vi "LSMcontroller_v64_updatedwaveformhandling.vi"() -> ()   [LabVIEW 2015] (continued)
                                frame False {
                                }
                                frame True {
                                n2579 = local write "set as Rp?"(FALSE ("set as Rp?")) -> ()
                                }
                              }
                            }
                          }
                        }
                        frame True {
                        }
                      }
                      n2580 = local read "sealtest"() -> (w5565:bool)
                      n2581 = Not(x=w5565) -> (.not. x?=w5564:bool)
                    }
                  }
                  frame #4 {
                    n2582 = call "tempconfigAO.vi"("command"="get") -> ("Temp Config out"=w5735:T25)  [unwired: 1 in]
                    n2583 = Unbundle By Name(w5735) -> ("AO"=w5734:refnum<k21>[], "E_AO"=w5733:errorcluster[])
                    n2584 = call "configuration.vi"("command"="get") -> ("config out"=w5716:T11)  [unwired: 2 in, 1 out]
                    n2585 = call "tempconfigAI.vi"("command"="get") -> ("Temp Config out"=w5722:T26)  [unwired: 1 in]
                    n2586 = Unbundle By Name(w5716) -> ("Device 1 sampleclock out"=w5713:tag, "Device 1 Starttrigger out"=w5712:tag)
                    n2587 = Unbundle By Name(w5722) -> ("AI"=w5723:refnum<k21>, "E_AI"=w5724:errorcluster)
                    n2588 = for {
                      tunnel: w5734 -> [w5739] mode=indexing
                      tunnel: w5733 -> [w5738] mode=indexing
                      tunnel: [w5737] -> w5729 mode=indexing
                      n2589 = call <vilib>:"DAQmx Stop Task.vi"("task/channels in"=w5739, "error in"=w5738) -> ("task out"=w5740:refnum<k21>, "error out"=w5741:errorcluster)  [unwired: 12 in]
                      n2590 = call <vilib>:"DAQmx Clear Task.vi"("task in"=w5740, "error in"=w5741) -> ("error out"=w5737:errorcluster)  [unwired: 13 in]
                    }
                    n2591 = call <vilib>:"DAQmx Stop Task.vi"("task/channels in"=w5723, "error in"=w5724) -> ("task out"=w5720:refnum<k21>, "error out"=w5719:errorcluster)  [unwired: 12 in]
                    n2592 = call <vilib>:"DAQmx Disconnect Terminals.vi"("source terminal"=tag "/Dev1/ai/SampleClock", "destination terminal"=w5713) -> ("error out"=w5710:errorcluster)  [unwired: 13 in]
                    n2593 = call <vilib>:"DAQmx Clear Task.vi"("task in"=w5720, "error in"=w5719) -> ("error out"=w5718:errorcluster)  [unwired: 13 in]
                    n2594 = call "tempconfigAO.vi"("command"="get") -> ("Temp Config out"=w5730:T25)  [unwired: 1 in]
                    n2595 = Bundle By Name(cluster=w5730, "E_AO"=w5729) -> (w5728:T25)
                    n2596 = call "tempconfigAI.vi"("command"="get") -> ("Temp Config out"=w5726:T26)  [unwired: 1 in]
                    n2597 = Bundle By Name(cluster=w5726, "E_AI"=w5718) -> (w5717:T26)
                    n2598 = call "tempconfigAO.vi"("Temp Config in"=w5728, "command"="set") -> ()  [unwired: 1 out]
                    n2599 = call <vilib>:"DAQmx Disconnect Terminals.vi"("source terminal"=tag "/Dev1/ai/StartTrigger", "destination terminal"=w5712, "error in"=w5710) -> ()  [unwired: 12 in, 1 out]
                    n2600 = call "tempconfigAI.vi"("Temp Config in"=w5717, "command"="set") -> ()  [unwired: 1 out]
                  }
                  frame #5 {
                    w5744 = T21 4 items=["no dialog", "OK message", "continue or stop message", "OK message + warnings", "continue/stop + warnings"] ("type of dialog (OK msg:1)")
                    n2601 = call "displayerrors.vi"() -> ("error IO"=w5743:errorcluster)
                    n2602 = call "zeropatch.vi"() -> ()  [unwired: 12 in]
                    n2603 = call <vilib>:"Simple Error Handler.vi"("type of dialog (OK msg:1)"=w5744, "error in (no error)"=w5743) -> ("error out"=w5742:errorcluster)  [unwired: 3 in, 4 out]
                    n2604 = call <vilib>:"Clear Errors.vi"("error in (no error)"=w5742) -> ()  [unwired: 5 in, 2 out]
                  }
                }
              }
            }
          }
          event "readpatch": Value Change {
            n2605 = event-data() -> ()  [unwired: 1 in, 6 out]
            n2606 = local read "readpatch"() -> (w5745:bool)
            n2607 = case shown="True" w5745 {
              frame False {
              }
              frame True {
                n2608 = stacked-sequence {
                  seq-local: [w5746 _ _ _ _ _] -> [_ w5779 _ w5831 _ _]
                  frame #0 {
                    n2609 = stacked-sequence {
                      tunnel: [_ w5758 _] -> w5746
                      frame #0 {
                        n2610 = call "2pparameters.vi"("command"="get") -> ("params out"=w5751:T10)  [unwired: 1 in]
                        n2611 = Unbundle By Name(w5751) -> ("autoshutter"=w5752:bool)
                        n2612 = local read "OCchecked?"() -> (w5749:bool)
                        n2613 = call "sealtestwfparams.vi"("command"="set") -> ()  [unwired: 6 in, 1 out]
                        n2614 = case shown="False" w5749 {
                          frame False {
                            n2615 = One Button Dialog(message="Is the OC gain correct?", button name ("OK")="ok") -> (true=w5753:bool)
                            n2616 = local write "OCchecked?"(w5753) -> ()
                          }
                          frame True {
                          }
                        }
                        n2617 = case shown="True" w5752 {
                          frame False {
                          }
                          frame True {
                            n2618 = call "shuttercontrol.vi"("command"="close") -> ()  [unwired: 1 in, 1 out]
                          }
                        }
                        n2619 = call "allAI-temp.vi"("command"=enum16{"get", "set", "clear", "append"}."clear") -> ()  [unwired: 3 in, 2 out]
                      }
                      frame #1 {
                        n2620 = call "sealtestwfparams.vi"("command"="get") -> ("Params out"=w5764:T22)  [unwired: 6 in]
                        n2621 = Unbundle By Name(w5764) -> ("AO parameters"=w5762:T23)
                        n2622 = Index Array(array=w5762, index=1) -> (element=w5761:T24)
                        n2623 = call "generateRampedSquareWave_fromAOparameters.vi"("AO params"=w5761) -> ("Waveform"=w5757:waveform(dbl), "wflength"=w5758:i32)
                        n2624 = Build Array(w5757) -> (w5760:waveform(dbl)[])
                        n2625 = call "waveformssealtestbuffer.vi"("AO wf in"=w5760, "command"="set") -> ()  [unwired: 1 out]
                      }
                      frame #2 {
                        n2626 = local read "Vholding (mV)"() -> (w5767:sgl)
                        n2627 = local read "Current Clamp"() -> (w5773:bool)
                        n2628 = local read "Voltage Clamp"() -> (w5772:bool)
                        n2629 = local read "OCgain"() -> (w5768:sgl)
                        n2630 = local read "CC_ICgain"() -> (w5771:dbl)
                        n2631 = local read "holdon"() -> (w5766:bool)
                        n2632 = call "patchparameters.vi"("command"="get") -> ("Params out"=w5775:T13)  [unwired: 1 in]
                        n2633 = Bundle By Name(cluster=w5775, "VC"=w5772, "CC"=w5773, "CC_icg (pA/mv)"=w5771, "VC_icg (mV/mV)"=10.0, "OCG (mV/pA)"=w5768, "OVG (mV/mV)"=0.1, "Vhold (mV)"=w5767, "holdon"=w5766) -> (w5774:T13)
                        n2634 = call "patchparameters.vi"("Params in"=w5774, "command"="set") -> ()  [unwired: 1 out]
                      }
                    }
                  }
                  frame #1 {
                    w5778 = 2
                    n2635 = call "patchparameters.vi"("command"="get") -> ("Params out"=w5786:T13)  [unwired: 1 in]
                    n2636 = Unbundle By Name(w5786) -> ("holdon"=w5785:bool, "Vhold (mV)"=w5784:sgl, "CC_icg (pA/mv)"=w5792:sgl, "CC"=w5790:bool, "VC_icg (mV/mV)"=w5791:sgl)
                    n2637 = Select(t=w5792, s=w5790, f=w5791) -> (s? t:f=w5793:sgl)
                    n2638 = To Single Precision Float(number=0.001 ("y")) -> (single precision float=w5794:sgl)
                    n2639 = Compound Arithmetic op=MULTIPLY(w5784, w5793, w5794) -> (w5788:sgl)
                    n2640 = case shown="False" w5785 {
                      tunnel: w5788 -> [_ w5806]
                      tunnel: [0.0 w5806] -> w5781
                      frame False {
                      }
                      frame True {
                      }
                    }
                    n2641 = Greater Than 0?(x=w5778) -> (x > 0?=w5780:bool)
                    n2642 = case shown="True" w5780 {
                      tunnel: w5779 -> [_ w5795]
                      tunnel: w5778 -> [_ w5798]
                      frame False {
                      }
                      frame True {
                        n2643 = Initialize Array(sgl 0.0 ("element"), w5798, w5795) -> (w5796:sgl[][])
                        n2644 = call "allAI-temp.vi"("array in"=w5796, "command"=enum16{"get", "set", "clear", "append"}."set") -> ()  [unwired: 2 in, 2 out]
                      }
                    }
                    n2645 = flat-sequence {
                      tunnel: w5779 -> [w5802]
                      tunnel: w5779 -> [w5801]
                      tunnel: [w5801] -> w5783
                      tunnel: [w5800] -> w5782
                      tunnel: w5781 -> [w5800]
                      tunnel: w5783 -> [w5804]
                      tunnel: w5782 -> [w5803]
                      frame #0 {
                        n2646 = call "prepAI_sealtest.vi"("samples per channel"=w5802) -> ()  [unwired: 2 in]
                      }
                      frame #1 {
                        n2647 = call "prepAO_sealtest.vi"("Vhold"=w5803, "samples per channel"=w5804) -> ()  [unwired: 1 in]
                      }
                    }
                  }
                  frame #2 {
                    n2648 = stacked-sequence {
                      frame #0 {
                        n2649 = call "tempconfigAO.vi"("command"="get") -> ("Temp Config out"=w5810:T25)  [unwired: 1 in]
                        n2650 = Unbundle By Name(w5810) -> ("AO"=w5811:refnum<k21>[], "E_AO"=w5812:errorcluster[])
                        n2651 = for {
                          tunnel: w5811 -> [w5820] mode=indexing
                          tunnel: w5812 -> [w5819] mode=indexing
                          tunnel: [w5818] -> w5814 mode=indexing
                          tunnel: [w5817] -> w5815 mode=indexing
                          n2652 = call <vilib>:"DAQmx Start Task.vi"("task/channels in"=w5820, "error in"=w5819) -> ("task out"=w5818:refnum<k21>, "error out"=w5817:errorcluster)  [unwired: 12 in]
                        }
                        n2653 = call "tempconfigAO.vi"("command"="get") -> ("Temp Config out"=w5813:T25)  [unwired: 1 in]
                        n2654 = Bundle By Name(cluster=w5813, "AO"=w5814, "E_AO"=w5815) -> (w5816:T25)
                        n2655 = call "tempconfigAO.vi"("Temp Config in"=w5816, "command"="set") -> ()  [unwired: 1 out]
                      }
                      frame #1 {
                        n2656 = call "tempconfigAI.vi"("command"="get") -> ("Temp Config out"=w5822:T26)  [unwired: 1 in]
                        n2657 = Unbundle By Name(w5822) -> ("AI"=w5827:refnum<k21>, "E_AI"=w5828:errorcluster)
                        n2658 = call <vilib>:"DAQmx Start Task.vi"("task/channels in"=w5827, "error in"=w5828) -> ("task out"=w5829:refnum<k21>, "error out"=w5830:errorcluster)  [unwired: 12 in]
                        n2659 = call "tempconfigAI.vi"("command"="get") -> ("Temp Config out"=w5824:T26)  [unwired: 1 in]
                        n2660 = Bundle By Name(cluster=w5824, "AI"=w5829, "E_AI"=w5830) -> (w5826:T26)
                        n2661 = call "tempconfigAI.vi"("Temp Config in"=w5826, "command"="set") -> ()  [unwired: 1 out]
                      }
                    }
                  }
                  frame #3 {
                    n2662 = while {
                      tunnel: w5831 -> [w5832]
                      stop <- w5833 stop-if-true
                      n2663 = local read "readpatch"() -> (w5836:bool)
                      n2664 = Not(x=w5836) -> (.not. x?=w5835:bool)
                      n2665 = case shown="True" w5835 {
                        tunnel: w5832 -> [w5837 _]
                        frame False {
                          n2666 = stacked-sequence {
                            seq-local: [w5838 _ _ _ _ _] -> [_ w5847 _ w5870 w5917 w5936]
                            tunnel: w5837 -> [_ _ w5855 _ w5916 _]
                            frame #0 {
                              n2667 = call "patchparameters.vi"("command"="get") -> ("Params out"=w5845:T13)  [unwired: 1 in]
                              n2668 = local read "Vholding (mV)"() -> (w5842:sgl)
                              n2669 = Unbundle By Name(w5845) -> ("Vhold (mV)"=w5841:sgl, "holdon"=w5844:bool)
                              n2670 = local read "holdon"() -> (w5843:bool)
                              n2671 = Not Equal?(x=w5842, y=w5841) -> (x != y?=w5840:bool)
                              n2672 = Not Equal?(x=w5844, y=w5843) -> (x != y?=w5839:bool)
                              n2673 = Or(x=w5840, y=w5839) -> (x .or. y?=w5838:bool)
                            }
                            frame #1 {
                              n2674 = case shown="False" w5847 {
                                frame False {
                                }
                                frame True {
                                n2675 = local read "Vholding (mV)"() -> (w5850:sgl)
                                n2676 = local read "holdon"() -> (w5848:bool)
                                n2677 = call "patchparameters.vi"("command"="get") -> ("Params out"=w5851:T13)  [unwired: 1 in]
                                n2678 = Bundle By Name(cluster=w5851, "Vhold (mV)"=w5850, "holdon"=w5848) -> (w5849:T13)
                                n2679 = call "patchparameters.vi"("Params in"=w5849, "command"="set") -> ()  [unwired: 1 out]
                                }
                              }
                            }
                            frame #2 {
                              n2680 = call "tempconfigAI.vi"("command"="get") -> ("Temp Config out"=w5865:T26)  [unwired: 1 in]
                              n2681 = Unbundle By Name(w5865) -> ("AI"=w5864:refnum<k21>, "E_AI"=w5863:errorcluster)
                              n2682 = call-poly <vilib>:"DAQmx Read.vi"("task/channels in"=w5864, "number of samples per channel"=w5855, "timeout"=10.0, "error in"=w5863) -> ("task out"=w5859:refnum<k21>, "data"=w5856:i16[][], "error out"=w5868:errorcluster)  [unwired: 9 in]
                              n2683 = call "tempconfigAI.vi"("command"="get") -> ("Temp Config out"=w5860:T26)  [unwired: 1 in]
                              n2684 = Bundle By Name(cluster=w5860, "AI"=w5859, "E_AI"=w5868) -> (w5867:T26)
                              n2685 = To Single Precision Float(number=w5856) -> (single precision float=w5858:sgl[][])
                              n2686 = call "tempconfigAI.vi"("Temp Config in"=w5867, "command"="set") -> ()  [unwired: 1 out]
                              n2687 = call "allAI-temp.vi"("array in"=w5858, "command"=enum16{"get", "set", "clear", "append"}."set") -> ()  [unwired: 2 in, 2 out]
                            }
                            frame #3 {
                              n2688 = case shown="True" w5870 {
                                frame False {
                                }
                                frame True {
                                n2689 = call "tempconfigAO.vi"("command"="get") -> ("Temp Config out"=w5909:T25)  [unwired: 1 in]
                                n2690 = Unbundle By Name(w5909) -> ("AO"=w5908:refnum<k21>[], "E_AO"=w5907:errorcluster[])
                                n2691 = call "tempconfigAI.vi"("command"="get") -> ("Temp Config out"=w5896:T26)  [unwired: 1 in]
                                n2692 = Unbundle By Name(w5896) -> ("AI"=w5897:refnum<k21>, "E_AI"=w5898:errorcluster)
                                n2693 = for {
                                tunnel: w5908 -> [w5913] mode=indexing
                                tunnel: w5907 -> [w5912] mode=indexing
                                tunnel: [w5911] -> w5903 mode=indexing
                                n2694 = call <vilib>:"DAQmx Stop Task.vi"("task/channels in"=w5913, "error in"=w5912) -> ("task out"=w5914:refnum<k21>, "error out"=w5915:errorcluster)  [unwired: 12 in]
                                n2695 = call <vilib>:"DAQmx Clear Task.vi"("task in"=w5914, "error in"=w5915) -> ("error out"=w5911:errorcluster)  [unwired: 13 in]
                                }
                                n2696 = call <vilib>:"DAQmx Stop Task.vi"("task/channels in"=w5897, "error in"=w5898) -> ("task out"=w5894:refnum<k21>, "error out"=w5893:errorcluster)  [unwired: 12 in]
                                n2697 = call <vilib>:"DAQmx Clear Task.vi"("task in"=w5894, "error in"=w5893) -> ("error out"=w5892:errorcluster)  [unwired: 13 in]
                                n2698 = call "tempconfigAO.vi"("command"="get") -> ("Temp Config out"=w5904:T25)  [unwired: 1 in]
                                n2699 = Bundle By Name(cluster=w5904, "E_AO"=w5903) -> (w5902:T25)
                                n2700 = call "tempconfigAI.vi"("command"="get") -> ("Temp Config out"=w5900:T26)  [unwired: 1 in]
                                n2701 = Bundle By Name(cluster=w5900, "E_AI"=w5892) -> (w5891:T26)
                                n2702 = call "tempconfigAO.vi"("Temp Config in"=w5902, "command"="set") -> ()  [unwired: 1 out]
                                n2703 = call "tempconfigAI.vi"("Temp Config in"=w5891, "command"="set") -> ()  [unwired: 1 out]
                                }
                              }
                              n2704 = call "allAI-temp.vi"("command"=enum16{"get", "set", "clear", "append"}."get") -> ("array out"=w5874:sgl[][])  [unwired: 3 in, 1 out]
                              n2705 = call "tempconfigAI.vi"("command"="get") -> ("Temp Config out"=w5886:T26)  [unwired: 1 in]
                              n2706 = call "tempconfigAI.vi"("command"="get") -> ("Temp Config out"=w5888:T26)  [unwired: 1 in]
                              n2707 = Unbundle By Name(w5886) -> ("header"=w5884:dbl[])
                              n2708 = Unbundle By Name(w5888) -> ("header"=w5890:dbl[])
                              n2709 = Index Array(array=w5874, index (row) #1=1 ("index (row)"), index (row) #2=0 ("index (row)")) -> (element #1=w5872:sgl[], element #2=w5871:sgl[])  [unwired: 2 in]
                              n2710 = local read "OCgain"() -> (w5878:sgl)
                              n2711 = call "Unscaledtoscaled.vi"("Unscaled Data"=w5872, "Header Information"=w5884) -> ("Array"=w5883:sgl[])  [unwired: 1 in]
                              n2712 = call "Unscaledtoscaled.vi"("Unscaled Data"=w5871, "Header Information"=w5890) -> ("Array"=w5887:sgl[])  [unwired: 1 in]
                              n2713 = Multiply(x=w5883, y=0.1) -> (x*y=w5880:dbl[])
                              n2714 = Divide(x=w5887, y=w5878) -> (x/y=w5879:sgl[])
                              n2715 = Build Array(w5880, w5879) -> (w5882:dbl[][])
                              n2716 = Multiply(x=w5882, y=1000.0) -> (x*y=w5869:dbl[][])
                              n2717 = local write "Patch readout"(w5869) -> ()
                            }
                            frame #4 {
                              n2718 = case shown="True" w5917 {
                                tunnel: w5916 -> [_ w5918]
                                frame False {
                                }
                                frame True {
                                n2719 = call "patchparameters.vi"("command"="get") -> ("Params out"=w5922:T13)  [unwired: 1 in]
                                n2720 = Unbundle By Name(w5922) -> ("holdon"=w5921:bool, "Vhold (mV)"=w5920:sgl, "CC_icg (pA/mv)"=w5928:sgl, "CC"=w5926:bool, "VC_icg (mV/mV)"=w5927:sgl)
                                n2721 = Select(t=w5928, s=w5926, f=w5927) -> (s? t:f=w5929:sgl)
                                n2722 = To Single Precision Float(number=0.001 ("y")) -> (single precision float=w5930:sgl)
                                n2723 = Compound Arithmetic op=MULTIPLY(w5920, w5929, w5930) -> (w5924:sgl)
                                n2724 = case shown="True" w5921 {
                                tunnel: w5924 -> [_ w5935]
                                tunnel: [0.0 w5935] -> w5919
                                frame False {
                                }
                                frame True {
                                }
                                }
                                n2725 = flat-sequence {
                                tunnel: w5918 -> [w5931]
                                tunnel: w5919 -> [w5933]
                                tunnel: w5918 -> [w5932]
                                frame #0 {
                                n2726 = call "prepAI_sealtest.vi"("samples per channel"=w5931) -> ()  [unwired: 2 in]
                                }
                                frame #1 {
                                n2727 = call "prepAO_sealtest.vi"("Vhold"=w5933, "samples per channel"=w5932) -> ()  [unwired: 1 in]
                                }
                                }
                                }
                              }
                            }
                            frame #5 {
                              n2728 = case shown="True" w5936 {
                                frame False {
                                }
                                frame True {
                                n2729 = stacked-sequence {
                                frame #0 {
                                n2730 = call "tempconfigAO.vi"("command"="get") -> ("Temp Config out"=w5943:T25)  [unwired: 1 in]
                                n2731 = Unbundle By Name(w5943) -> ("AO"=w5942:refnum<k21>[], "E_AO"=w5941:errorcluster[])
                                n2732 = for {
                                tunnel: w5942 -> [w5950] mode=indexing
                                tunnel: w5941 -> [w5949] mode=indexing
                                tunnel: [w5948] -> w5939 mode=indexing
                                tunnel: [w5947] -> w5938 mode=indexing
                                n2733 = call <vilib>:"DAQmx Start Task.vi"("task/channels in"=w5950, "error in"=w5949) -> ("task out"=w5948:refnum<k21>, "error out"=w5947:errorcluster)  [unwired: 12 in]
                                }
                                n2734 = call "tempconfigAO.vi"("command"="get") -> ("Temp Config out"=w5940:T25)  [unwired: 1 in]
                                n2735 = Bundle By Name(cluster=w5940, "AO"=w5939, "E_AO"=w5938) -> (w5937:T25)
                                n2736 = call "tempconfigAO.vi"("Temp Config in"=w5937, "command"="set") -> ()  [unwired: 1 out]
                                }
                                frame #1 {
                                n2737 = call "tempconfigAI.vi"("command"="get") -> ("Temp Config out"=w5952:T26)  [unwired: 1 in]
                                n2738 = Unbundle By Name(w5952) -> ("AI"=w5957:refnum<k21>, "E_AI"=w5958:errorcluster)
                                n2739 = call <vilib>:"DAQmx Start Task.vi"("task/channels in"=w5957, "error in"=w5958) -> ("task out"=w5959:refnum<k21>, "error out"=w5960:errorcluster)  [unwired: 12 in]
                                n2740 = call "tempconfigAI.vi"("command"="get") -> ("Temp Config out"=w5954:T26)  [unwired: 1 in]
                                n2741 = Bundle By Name(cluster=w5954, "AI"=w5959, "E_AI"=w5960) -> (w5956:T26)
                                n2742 = call "tempconfigAI.vi"("Temp Config in"=w5956, "command"="set") -> ()  [unwired: 1 out]
                                }
                                }
                                }
                              }
                            }
                          }
                        }
                        frame True {
                        }
                      }
                      n2743 = local read "readpatch"() -> (w5834:bool)
                      n2744 = Not(x=w5834) -> (.not. x?=w5833:bool)
                    }
                  }
                  frame #4 {
                    n2745 = call "tempconfigAO.vi"("command"="get") -> ("Temp Config out"=w5986:T25)  [unwired: 1 in]
                    n2746 = Unbundle By Name(w5986) -> ("AO"=w5985:refnum<k21>[], "E_AO"=w5984:errorcluster[])
                    n2747 = call "configuration.vi"("command"="get") -> ("config out"=w5967:T11)  [unwired: 2 in, 1 out]
                    n2748 = call "tempconfigAI.vi"("command"="get") -> ("Temp Config out"=w5973:T26)  [unwired: 1 in]
                    n2749 = Unbundle By Name(w5967) -> ("Device 1 sampleclock out"=w5964:tag, "Device 1 Starttrigger out"=w5963:tag)
                    n2750 = Unbundle By Name(w5973) -> ("AI"=w5974:refnum<k21>, "E_AI"=w5975:errorcluster)
                    n2751 = for {
                      tunnel: w5985 -> [w5990] mode=indexing
                      tunnel: w5984 -> [w5989] mode=indexing
                      tunnel: [w5988] -> w5980 mode=indexing
                      n2752 = call <vilib>:"DAQmx Stop Task.vi"("task/channels in"=w5990, "error in"=w5989) -> ("task out"=w5991:refnum<k21>, "error out"=w5992:errorcluster)  [unwired: 12 in]
                      n2753 = call <vilib>:"DAQmx Clear Task.vi"("task in"=w5991, "error in"=w5992) -> ("error out"=w5988:errorcluster)  [unwired: 13 in]
                    }
                    n2754 = call <vilib>:"DAQmx Stop Task.vi"("task/channels in"=w5974, "error in"=w5975) -> ("task out"=w5971:refnum<k21>, "error out"=w5970:errorcluster)  [unwired: 12 in]
                    n2755 = call <vilib>:"DAQmx Disconnect Terminals.vi"("source terminal"=tag "/Dev1/ai/SampleClock", "destination terminal"=w5964) -> ("error out"=w5961:errorcluster)  [unwired: 13 in]
                    n2756 = call <vilib>:"DAQmx Clear Task.vi"("task in"=w5971, "error in"=w5970) -> ("error out"=w5969:errorcluster)  [unwired: 13 in]
                    n2757 = call "tempconfigAO.vi"("command"="get") -> ("Temp Config out"=w5981:T25)  [unwired: 1 in]
                    n2758 = Bundle By Name(cluster=w5981, "E_AO"=w5980) -> (w5979:T25)
                    n2759 = call "tempconfigAI.vi"("command"="get") -> ("Temp Config out"=w5977:T26)  [unwired: 1 in]
                    n2760 = Bundle By Name(cluster=w5977, "E_AI"=w5969) -> (w5968:T26)
                    n2761 = call "tempconfigAO.vi"("Temp Config in"=w5979, "command"="set") -> ()  [unwired: 1 out]
                    n2762 = call <vilib>:"DAQmx Disconnect Terminals.vi"("source terminal"=tag "/Dev1/ai/StartTrigger", "destination terminal"=w5963, "error in"=w5961) -> ()  [unwired: 12 in, 1 out]
                    n2763 = call "tempconfigAI.vi"("Temp Config in"=w5968, "command"="set") -> ()  [unwired: 1 out]
                  }
                  frame #5 {
                    w5995 = T21 4 items=["no dialog", "OK message", "continue or stop message", "OK message + warnings", "continue/stop + warnings"] ("type of dialog (OK msg:1)")
                    n2764 = call "displayerrors.vi"() -> ("error IO"=w5994:errorcluster)
                    n2765 = call "zeropatch.vi"() -> ()  [unwired: 12 in]
                    n2766 = call <vilib>:"Simple Error Handler.vi"("type of dialog (OK msg:1)"=w5995, "error in (no error)"=w5994) -> ("error out"=w5993:errorcluster)  [unwired: 3 in, 4 out]
                    n2767 = call <vilib>:"Clear Errors.vi"("error in (no error)"=w5993) -> ()  [unwired: 5 in, 2 out]
                  }
                }
              }
            }
          }
          event "Current Clamp": Value Change {
            n2768 = event-data() -> ()  [unwired: 1 in, 6 out]
            n2769 = local read "Current Clamp"() -> (w6000:bool)
            n2770 = property on="Vholding (mV)" class="DigNum (strict)"("Caption.Text"="Ihold (pA)") -> ()  [unwired: 2 in, 2 out]
            n2771 = Not(x=w6000) -> (.not. x?=w5999:bool)
            n2772 = property on="Voltage Clamp" class="Bool (strict)"("Value"=w5999) -> ()  [unwired: 2 in, 2 out]
            n2773 = One Button Dialog(message="Have you switched the HEKA to CC and changed the external input cable?", button name ("OK")="Ok") -> ()  [unwired: 1 out]
          }
          event "Voltage Clamp": Value Change {
            n2774 = event-data() -> ()  [unwired: 1 in, 6 out]
            n2775 = local read "Voltage Clamp"() -> (w6005:bool)
            n2776 = Not(x=w6005) -> (.not. x?=w6004:bool)
            n2777 = property on="Current Clamp" class="Bool (strict)"("Value"=w6004) -> ()  [unwired: 2 in, 2 out]
            n2778 = One Button Dialog(message="Have you switched the HEKA to VC and changed the external input cable?", button name ("OK")="Ok") -> ()  [unwired: 1 out]
            n2779 = property on="Vholding (mV)" class="DigNum (strict)"("Caption.Text"="Vhold (mV)") -> ()  [unwired: 2 in, 2 out]
          }
          event "OCgain": Value Change {
            n2780 = event-data() -> ()  [unwired: 1 in, 6 out]
            n2781 = local read "OCgain"() -> (w6008:sgl)
            n2782 = Less?(x=w6008, y=0.3) -> (x < y?=w6006:bool)
            n2783 = case shown="True" w6006 {
              frame False {
                w6009 = 10.0 items=["0.1"=10.0, "10"=0.1] ("CC_ICgain")
                n2784 = local write "CC_ICgain"(w6009) -> ()
              }
              frame True {
                w6010 = 0.1 items=["0.1"=10.0, "10"=0.1] ("CC_ICgain")
                n2785 = local write "CC_ICgain"(w6010) -> ()
              }
            }
          }
          event "holdon": Value Change {
            n2786 = event-data() -> ()  [unwired: 1 in, 6 out]
            n2787 = stacked-sequence {
              frame #0 {
                n2788 = local read "Vholding (mV)"() -> (w6014:sgl)
                n2789 = local read "holdon"() -> (w6011:bool)
                n2790 = call "patchparameters.vi"("command"="get") -> ("Params out"=w6015:T13)  [unwired: 1 in]
                n2791 = Bundle By Name(cluster=w6015, "Vhold (mV)"=w6014, "holdon"=w6011) -> (w6012:T13)
                n2792 = call "patchparameters.vi"("Params in"=w6012, "command"="set") -> ()  [unwired: 1 out]
              }
              frame #1 {
                n2793 = call "zeropatch.vi"() -> ()  [unwired: 12 in]
              }
            }
          }
          event "Vholding (mV)": Value Change {
            n2794 = event-data() -> ()  [unwired: 1 in, 6 out]
            n2795 = local read "holdon"() -> (w6017:bool)
            n2796 = case shown="True" w6017 {
              frame False {
              }
              frame True {
                n2797 = stacked-sequence {
                  frame #0 {
                    n2798 = local read "Vholding (mV)"() -> (w6020:sgl)
                    n2799 = local read "holdon"() -> (w6021:bool)
                    n2800 = call "patchparameters.vi"("command"="get") -> ("Params out"=w6022:T13)  [unwired: 1 in]
                    n2801 = Bundle By Name(cluster=w6022, "Vhold (mV)"=w6020, "holdon"=w6021) -> (w6018:T13)
                    n2802 = call "patchparameters.vi"("Params in"=w6018, "command"="set") -> ()  [unwired: 1 out]
                  }
                  frame #1 {
                    n2803 = call "zeropatch.vi"() -> ()  [unwired: 12 in]
                  }
                }
              }
            }
          }
          event "AI channels": Value Change {
            n2804 = event-data() -> ()  [unwired: 1 in, 6 out]
            n2805 = local read "CI channels"() -> (w6031:i32[])
            n2806 = local read "AI channels"() -> (w6032:i32[])
            n2807 = call "configuration.vi"("command"="get") -> ("config out"=w6025:T11)  [unwired: 2 in, 1 out]
            n2808 = Unbundle By Name(w6025) -> ("CI names"=w6026:string[], "AI names"=w6027:string[])
            n2809 = for {
              tunnel: w6031 -> [w6037] mode=indexing
              tunnel: w6026 -> [w6038]
              tunnel: [w6036] -> w6028 mode=indexing
              n2810 = Index Array(array=w6038, index=w6037) -> (element=w6036:string)
            }
            n2811 = for {
              tunnel: w6032 -> [w6034] mode=indexing
              tunnel: w6027 -> [w6035]
              tunnel: [w6033] -> w6029 mode=indexing
              n2812 = Index Array(array=w6035, index=w6034) -> (element=w6033:string)
            }
            n2813 = Build Array (concatenate)(w6028, w6029) -> (w6030:string[])
            n2814 = property on="image1list" class="Ring (strict)"("Strings []"=w6030) -> ()  [unwired: 2 in, 2 out]
            n2815 = property on="image2list" class="Ring (strict)"("Strings []"=w6030) -> ()  [unwired: 2 in, 2 out]
          }
          event "CI channels": Value Change {
            n2816 = event-data() -> ()  [unwired: 1 in, 6 out]
            n2817 = local read "CI channels"() -> (w6046:i32[])
            n2818 = local read "AI channels"() -> (w6047:i32[])
            n2819 = call "configuration.vi"("command"="get") -> ("config out"=w6040:T11)  [unwired: 2 in, 1 out]
            n2820 = Unbundle By Name(w6040) -> ("CI names"=w6041:string[], "AI names"=w6042:string[])
            n2821 = for {
              tunnel: w6046 -> [w6052] mode=indexing
              tunnel: w6041 -> [w6053]
              tunnel: [w6051] -> w6043 mode=indexing
              n2822 = Index Array(array=w6053, index=w6052) -> (element=w6051:string)
            }
            n2823 = for {
              tunnel: w6047 -> [w6049] mode=indexing
              tunnel: w6042 -> [w6050]
              tunnel: [w6048] -> w6044 mode=indexing
              n2824 = Index Array(array=w6050, index=w6049) -> (element=w6048:string)
            }
            n2825 = Build Array (concatenate)(w6043, w6044) -> (w6045:string[])
            n2826 = property on="image1list" class="Ring (strict)"("Strings []"=w6045) -> ()  [unwired: 2 in, 2 out]
            n2827 = property on="image2list" class="Ring (strict)"("Strings []"=w6045) -> ()  [unwired: 2 in, 2 out]
          }
          event "setdatdir": Value Change {
            n2828 = event-data() -> ()  [unwired: 1 in, 5 out]
            n2829 = case shown="True" "setdatdir" {
              frame False {
              }
              frame True {
                n2830 = stacked-sequence {
                  frame #0 {
                    n2831 = local read "data dir"() -> (w6055:path)
                    n2832 = call "File Dialog"("start path"=w6055, "prompt"="Please select data directory...") -> ("selected path"=w6057:path, "cancelled"=w6056:bool, "error out"=w6058:errorcluster)  [unwired: 10 in, 1 out]
                    n2833 = case shown="False" w6056 {
                      tunnel: w6057 -> [w6066 _]
                      tunnel: w6058 -> [w6063 w6069]
                      tunnel: [w6061 w6069] -> w6060
                      frame False {
                        n2834 = local write "data dir"(w6066) -> ()
                        n2835 = call "configuration.vi"("error in"=w6063, "command"="get") -> ("Error out"=w6062:errorcluster, "config out"=w6068:T11)  [unwired: 1 in]
                        n2836 = Bundle By Name(cluster=w6068, "master data dir"=w6066) -> (w6067:T11)
                        n2837 = call "configuration.vi"("error in"=w6062, "config in"=w6067, "command"="set") -> ("Error out"=w6061:errorcluster)  [unwired: 1 out]
                      }
                      frame True {
                      }
                    }
                    n2838 = local write "status"(w6060) -> ()
                  }
                  frame #1 {
                    n2839 = property on="setdatdir" class="Bool (strict)"("Value"=FALSE ("setdatdir")) -> ()  [unwired: 2 in, 2 out]
                  }
                }
              }
            }
          }
          event "Shutter": Value Change {
            n2840 = event-data() -> ()  [unwired: 1 in, 5 out]
            n2841 = case shown="False" "Shutter" {
              frame False {
                n2842 = call "shuttercontrol.vi"("command"="close") -> ()  [unwired: 1 in, 1 out]
              }
              frame True {
                n2843 = call "shuttercontrol.vi"("command"="open") -> ()  [unwired: 1 in, 1 out]
              }
            }
          }
          event "ROI": Value Change {
            n2844 = event-data() -> ()  [unwired: 1 in, 5 out]
            n2845 = local read "ROI"() -> (w6074:bool)
            n2846 = case shown="True" w6074 {
              frame False {
              }
              frame True {
                n2847 = stacked-sequence {
                  frame #0 {
                    n2848 = local read "Square pixels"() -> (w6091:bool)
                    n2849 = local read "square matrix"() -> (w6090:bool)
                    n2850 = local read "Vx-max ref"() -> (w6096:dbl)
                    n2851 = local read "Vx-min ref"() -> (w6095:dbl)
                    n2852 = local read "Vy-min ref"() -> (w6092:dbl)
                    n2853 = local read "ypixels ref"() -> (w6094:i32)
                    n2854 = local read "Vy-max ref"() -> (w6093:dbl)
                    n2855 = local read "xpixels ref"() -> (w6097:i32)
                    n2856 = local read "Angle ref"() -> (w6089:dbl)
                    n2857 = local read "Colormap"() -> (w6098:i32)
                    n2858 = call "2pparameters.vi"("command"="get") -> ("params out"=w6101:T10)  [unwired: 1 in]
                    n2859 = Bundle By Name(cluster=w6101, "Xpixels Img"=w6097, "Vx-min Img"=w6095, "VX-max Img"=w6096, "Ypixels Img"=w6094, "Vy-min Img"=w6092, "Vy-max Img"=w6093, "Colormap"=w6098, "square pixels"=w6091, "square matrix"=w6090, "Angle Img"=w6089) -> (w6100:T10)
                    n2860 = call "2pparameters.vi"("Params in"=w6100, "command"="set") -> ()  [unwired: 1 out]
                    n2861 = local read "Vx-max draw"() -> (w6081:dbl)
                    n2862 = local read "Angle drawing"() -> (w6088:dbl)
                    n2863 = local read "Vx-min draw"() -> (w6082:dbl)
                    n2864 = local read "Vy-min draw"() -> (w6085:dbl)
                    n2865 = local read "ypixels draw"() -> (w6083:dbl)
                    n2866 = local read "Vy-max draw"() -> (w6084:dbl)
                    n2867 = local read "Square pixels"() -> (w6086:bool)
                    n2868 = local read "square matrix"() -> (w6087:bool)
                    n2869 = local read "xpixels draw"() -> (w6080:dbl)
                    n2870 = local read "Colormap"() -> (w6079:i32)
                    n2871 = call "2pparameters.vi"("command"="get") -> ("params out"=w6076:T10)  [unwired: 1 in]
                    n2872 = Bundle By Name(cluster=w6076, "Xpixels"=w6080, "Vxminref"=w6082, "Vxmaxref"=w6081, "Ypixels"=w6083, "Vyminref"=w6085, "Vymaxref"=w6084, "Colormap"=w6079, "square pixels"=w6086, "square matrix"=w6087, "Angle draw"=w6088) -> (w6077:T10)
                    n2873 = call "2pparameters.vi"("Params in"=w6077, "command"="set") -> ()  [unwired: 1 out]
                  }
                  frame #1 {
                    n2874 = Current VI's Path() -> (path=w6112:path)
                    n2875 = Strip Path(path=w6112) -> (stripped path=w6113:path)  [unwired: 1 out]
                    n2876 = Build Path(base path=w6113, name or relative path="subVIs\\Image\\SetROI_v4.vi") -> (appended path=w6111:path)
                    n2877 = call <vilib>:"Set Busy.vi"() -> ("error out"=w6109:errorcluster)  [unwired: 10 in, 1 out]
                    n2878 = Open VI Reference(type specifier VI Refnum (for type only)=refnum<vi> refnum, vi path=w6111, error in (no error)=w6109) -> (vi reference=w6107:refnum<vi>, error out=w6105:errorcluster)  [unwired: 3 in]
                    n2879 = call-by-ref "?"(reference=w6107, error in=w6105) -> (reference out=w6106:refnum<vi>, error out=w6104:errorcluster)  [unwired: 1 in]
                    n2880 = Close Reference(reference=w6106, error in (no error)=w6104) -> (error out=w6108:errorcluster)
                    n2881 = call <vilib>:"Unset Busy.vi"("error in (no error)"=w6108) -> ()  [unwired: 10 in, 1 out]
                    n2882 = local write "status"(w6108) -> ()
                  }
                  frame #2 {
                    n2883 = call "2pparameters.vi"("command"="get") -> ("params out"=w6138:T10)  [unwired: 1 in]
                    n2884 = Unbundle By Name(w6138) -> ("Xpixels Img"=w6137:i32, "Vx-min Img"=w6136:dbl, "VX-max Img"=w6135:dbl, "Ypixels Img"=w6134:i32, "Vy-min Img"=w6133:dbl, "Vy-max Img"=w6132:dbl, "Colormap"=w6131:u16, "square pixels"=w6130:bool, "square matrix"=w6129:bool, "Angle Img"=w6128:dbl, "Drawing Mode"=w6127:u16)
                    n2885 = local write "xpixels ref"(w6137) -> ()
                    n2886 = local write "Vx-min ref"(w6136) -> ()
                    n2887 = local write "Vx-max ref"(w6135) -> ()
                    n2888 = local write "ypixels ref"(w6134) -> ()
                    n2889 = local write "Vy-min ref"(w6133) -> ()
                    n2890 = local write "Vy-max ref"(w6132) -> ()
                    n2891 = local write "Colormap"(w6131) -> ()
                    n2892 = local write "Square pixels"(w6130) -> ()
                    n2893 = local write "square matrix"(w6129) -> ()
                    n2894 = local write "Angle ref"(w6128) -> ()
                    n2895 = local write "ROI Type"(w6127) -> ()
                    n2896 = call "2pparameters.vi"("command"="get") -> ("params out"=w6121:T10)  [unwired: 1 in]
                    n2897 = Unbundle By Name(w6121) -> ("Xpixels"=w6115:i32, "Vxminref"=w6119:dbl, "Vxmaxref"=w6118:dbl, "Ypixels"=w6114:i32, "Vyminref"=w6117:dbl, "Vymaxref"=w6116:dbl, "Colormap"=w6122:u16, "square pixels"=w6123:bool, "square matrix"=w6124:bool, "Angle draw"=w6125:dbl, "Drawing Mode"=w6126:u16)
                    n2898 = local write "Vy-max draw"(w6116) -> ()
                    n2899 = local write "Angle drawing"(w6125) -> ()
                    n2900 = local write "Colormap"(w6122) -> ()
                    n2901 = local write "Square pixels"(w6123) -> ()
                    n2902 = local write "square matrix"(w6124) -> ()
                    n2903 = local write "ROI Type"(w6126) -> ()
                    n2904 = local write "xpixels draw"(w6115) -> ()
                    n2905 = local write "ypixels draw"(w6114) -> ()
                    n2906 = local write "Vx-min draw"(w6119) -> ()
                    n2907 = local write "Vx-max draw"(w6118) -> ()
                    n2908 = local write "Vy-min draw"(w6117) -> ()
                  }
                  frame #3 {
                    n2909 = property on="ROI" class="Bool (strict)"("Val(Sgnl)"=FALSE ("x/y scan")) -> ()  [unwired: 2 in, 2 out]
                  }
                }
              }
            }
          }
          event "Xdattype": Value Change {
            n2910 = event-data() -> ()  [unwired: 1 in, 1 out]
            n2911 = case shown="True" "Xdattype" {
              frame False {
              }
              frame True {
                n2912 = stacked-sequence {
                  frame #0 {
                    n2913 = Current VI's Path() -> (path=w6151:path)
                    n2914 = Strip Path(path=w6151) -> (stripped path=w6152:path)  [unwired: 1 out]
                    n2915 = Build Path(base path=w6152, name or relative path="subVIs\\Misc\\Changedataconfig.vi") -> (appended path=w6150:path)
                    n2916 = call <vilib>:"Set Busy.vi"() -> ("error out"=w6148:errorcluster)  [unwired: 10 in, 1 out]
                    n2917 = Open VI Reference(type specifier VI Refnum (for type only)=refnum<vi> refnum, vi path=w6150, error in (no error)=w6148) -> (vi reference=w6143:refnum<vi>, error out=w6145:errorcluster)  [unwired: 3 in]
                    n2918 = call-by-ref "?"(reference=w6143, error in=w6145) -> (reference out=w6147:refnum<vi>, error out=w6146:errorcluster)  [unwired: 12 in]
                    n2919 = Close Reference(reference=w6147, error in (no error)=w6146) -> (error out=w6142:errorcluster)
                    "status" <- w6142
                    n2920 = call <vilib>:"Unset Busy.vi"("error in (no error)"=w6142) -> ()  [unwired: 10 in, 1 out]
                  }
                  frame #1 {
                    n2921 = property on="Xdattype" class="Bool (strict)"("Val(Sgnl)"=FALSE ("x/y scan")) -> ()  [unwired: 2 in, 2 out]
                  }
                }
              }
            }
          }
          event "XautoOD": Value Change {
            n2922 = event-data() -> ()  [unwired: 1 in, 1 out]
            n2923 = case shown="True" "XautoOD" {
              frame False {
              }
              frame True {
                n2924 = stacked-sequence {
                  frame #0 {
                    n2925 = Current VI's Path() -> (path=w6164:path)
                    n2926 = Strip Path(path=w6164) -> (stripped path=w6165:path)  [unwired: 1 out]
                    n2927 = Build Path(base path=w6165, name or relative path="subVIs\\Misc\\ChangeautoODs.vi") -> (appended path=w6163:path)
                    n2928 = call <vilib>:"Set Busy.vi"() -> ("error out"=w6161:errorcluster)  [unwired: 10 in, 1 out]
                    n2929 = Open VI Reference(type specifier VI Refnum (for type only)=refnum<vi> refnum, vi path=w6163, error in (no error)=w6161) -> (vi reference=w6156:refnum<vi>, error out=w6158:errorcluster)  [unwired: 3 in]
                    n2930 = call-by-ref "?"(reference=w6156, error in=w6158) -> (reference out=w6160:refnum<vi>, error out=w6159:errorcluster)  [unwired: 12 in]
                    n2931 = Close Reference(reference=w6160, error in (no error)=w6159) -> (error out=w6155:errorcluster)
                    "status 2" <- w6155
                    n2932 = call <vilib>:"Unset Busy.vi"("error in (no error)"=w6155) -> ()  [unwired: 10 in, 1 out]
                  }
                  frame #1 {
                    n2933 = property on="XautoOD" class="Bool (strict)"("Val(Sgnl)"=FALSE ("x/y scan")) -> ()  [unwired: 2 in, 2 out]
                  }
                }
              }
            }
          }
          event "SetMan": Value Change {
            n2934 = event-data() -> ()  [unwired: 1 in, 1 out]
            n2935 = case shown="True" "SetMan" {
              frame False {
              }
              frame True {
                n2936 = stacked-sequence {
                  frame #0 {
                    w6168 = u16 0 items=["Rectangle", "Circle", "Freeform Boundary", "Freeform Interior"] ("ROI Type")
                    n2937 = local write "ROI Type"(w6168) -> ()
                    n2938 = local read "Square pixels"() -> (w6174:bool)
                    n2939 = case shown="True" w6174 {
                      frame False {
                        n2940 = local read "square matrix"() -> (w6175:bool)
                        n2941 = case shown="False" w6175 {
                          frame False {
                            "ypixels ref" <- "ypixels"
                            "xpixels ref" <- "xpixels"
                          }
                          frame True {
                            n2942 = local read "xpixels"() -> (w6180:i32)
                            n2943 = local read "ypixels"() -> (w6179:i32)
                            n2944 = Max & Min(x=w6180, y=w6179) -> (max(x,y)=w6178:i32)  [unwired: 1 out]
                            n2945 = local write "xpixels ref"(w6178) -> ()
                            n2946 = local write "ypixels ref"(w6178) -> ()
                          }
                        }
                      }
                      frame True {
                        n2947 = local read "square matrix"() -> (w6181:bool)
                        n2948 = case shown="False" w6181 {
                          frame False {
                            n2949 = local read "Vxmax"() -> (w6195:dbl)
                            n2950 = local read "Vx-min"() -> (w6194:dbl)
                            n2951 = local read "Vy-max"() -> (w6190:dbl)
                            n2952 = local read "Vy-min"() -> (w6191:dbl)
                            n2953 = Subtract(x=w6190, y=w6191) -> (x-y=w6192:dbl)
                            n2954 = Subtract(x=w6195, y=w6194) -> (x-y=w6193:dbl)
                            n2955 = Absolute Value(x=w6192) -> (abs(x)=w6183:dbl)
                            n2956 = Absolute Value(x=w6193) -> (abs(x)=w6184:dbl)
                            n2957 = Divide(x=w6184, y=w6183) -> (x/y=w6189:dbl)
                            n2958 = Greater Or Equal?(x=w6184, y=w6183) -> (x >= y?=w6182:bool)
                            n2959 = local read "xpixels"() -> (w6188:i32)
                            n2960 = local read "ypixels"() -> (w6185:i32)
                            n2961 = case shown="False" w6182 {
                              tunnel: w6189 -> [w6200 w6203]
                              tunnel: w6188 -> [w6197 _]
                              tunnel: [w6197 w6202] -> w6187
                              tunnel: [w6196 w6201] -> w6186
                              tunnel: w6185 -> [_ w6201]
                              frame False {
                                n2962 = To Double Precision Float(number=w6197) -> (double precision float=w6199:dbl)
                                n2963 = Divide(x=w6199, y=w6200) -> (x/y=w6198:dbl)
                                n2964 = To Long Integer(number=w6198) -> (32bit integer=w6196:i32)
                              }
                              frame True {
                                n2965 = To Double Precision Float(number=w6201) -> (double precision float=w6205:dbl)
                                n2966 = Multiply(x=w6205, y=w6203) -> (x*y=w6204:dbl)
                                n2967 = To Long Integer(number=w6204) -> (32bit integer=w6202:i32)
                              }
                            }
                            n2968 = local write "ypixels ref"(w6186) -> ()
                            n2969 = local write "xpixels ref"(w6187) -> ()
                          }
                          frame True {
                          }
                        }
                      }
                    }
                    "Vx-max ref" <- "Vxmax"
                    "Vx-min ref" <- "Vx-min"
                    "Vy-max ref" <- "Vy-max"
                    "Vy-min ref" <- "Vy-min"
                    "Angle ref" <- "Angle"
                  }
                  frame #1 {
                    n2970 = property on="SetMan" class="Bool (strict)"("Val(Sgnl)"=FALSE ("Value (Signaling)")) -> ()  [unwired: 2 in, 2 out]
                  }
                }
              }
            }
          }
          event "SetMan 2": Value Change {
            n2971 = event-data() -> ()  [unwired: 1 in, 1 out]
            n2972 = case shown="True" "SetMan 2" {
              frame False {
              }
              frame True {
                n2973 = stacked-sequence {
                  frame #0 {
                    n2974 = local write "Vx-ref"("Vx") -> ()
                    n2975 = local write "Vy-ref"("Vy") -> ()
                  }
                  frame #1 {
                    n2976 = property on="SetMan 2" class="Bool (strict)"("Val(Sgnl)"=FALSE ("Value (Signaling)")) -> ()  [unwired: 2 in, 2 out]
                  }
                }
              }
            }
          }
          event "Reset Coords": Value Change {
            n2977 = event-data() -> ("NewVal"=w6211:bool)  [unwired: 1 in, 5 out]
            n2978 = case shown="True" w6211 {
              frame False {
              }
              frame True {
                n2979 = stacked-sequence {
                  frame #0 {
                    n2980 = local write "xpixels"(256 ("xpixels")) -> ()
                    n2981 = local write "ypixels"(256 ("ypixels")) -> ()
                    n2982 = local write "Vxmax"(9.0 ("Vx-max")) -> ()
                    n2983 = local write "Vx-min"(-9.0 ("Vx-min")) -> ()
                    n2984 = local write "Vy-max"(9.0 ("Vy-max")) -> ()
                    n2985 = local write "Vy-min"(-9.0 ("Vy-min")) -> ()
                    n2986 = local write "Angle"(0.0 ("Angle")) -> ()
                  }
                  frame #1 {
                    n2987 = property on="Reset Coords" class="Bool (strict)"("Value"=FALSE ("TROI")) -> ()  [unwired: 2 in, 2 out]
                  }
                }
              }
            }
          }
          event "TROI": Value Change {
            n2988 = event-data() -> ()  [unwired: 1 in, 1 out]
            n2989 = case shown="True" "TROI" {
              frame False {
              }
              frame True {
                n2990 = stacked-sequence {
                  frame #0 {
                    n2991 = local read "Vy-min ref"() -> (w6225:dbl)
                    n2992 = local read "Vy-max ref"() -> (w6224:dbl)
                    n2993 = local read "Vx-max ref"() -> (w6222:dbl)
                    n2994 = local read "Vx-min ref"() -> (w6223:dbl)
                    n2995 = local read "ypixels ref"() -> (w6227:i32)
                    n2996 = local read "xpixels ref"() -> (w6226:i32)
                    n2997 = local read "Angle ref"() -> (w6221:dbl)
                    n2998 = local write "Angle"(w6221) -> ()
                    n2999 = local write "xpixels"(w6226) -> ()
                    n3000 = local write "Vy-min"(w6225) -> ()
                    n3001 = local write "Vy-max"(w6224) -> ()
                    n3002 = local write "Vx-min"(w6223) -> ()
                    n3003 = local write "ypixels"(w6227) -> ()
                    n3004 = local write "Vxmax"(w6222) -> ()
                  }
                  frame #1 {
                    n3005 = property on="TROI" class="Bool (strict)"("Value"=FALSE ("TROI")) -> ()  [unwired: 2 in, 2 out]
                  }
                }
              }
            }
          }
          event "TROI 2": Value Change {
            n3006 = event-data() -> ()  [unwired: 1 in, 1 out]
            n3007 = case shown="True" "TROI 2" {
              frame False {
              }
              frame True {
                n3008 = stacked-sequence {
                  frame #0 {
                    n3009 = local read "Vx-ref"() -> (w6230:dbl)
                    n3010 = local read "Vy-ref"() -> (w6231:dbl)
                    n3011 = local write "Vx"(w6230) -> ()
                    n3012 = local write "Vy"(w6231) -> ()
                  }
                  frame #1 {
                    n3013 = property on="TROI 2" class="Bool (strict)"("Value"=FALSE ("TROI")) -> ()  [unwired: 2 in, 2 out]
                  }
                }
              }
            }
          }
          event "Square pixels": Value Change {
            n3014 = event-data() -> ()  [unwired: 1 in, 1 out]
            n3015 = case shown="True" "Square pixels" {
              frame False {
              }
              frame True {
                n3016 = property on="square matrix" class="Bool (strict)"("Value"=FALSE ("square matrix")) -> ()  [unwired: 2 in, 2 out]
                n3017 = property on="Square pixels" class="Bool (strict)"("Value"=TRUE ("square matrix")) -> ()  [unwired: 2 in, 2 out]
              }
            }
          }
          event "square matrix": Value Change {
            n3018 = event-data() -> ()  [unwired: 1 in, 1 out]
            n3019 = case shown="True" "square matrix" {
              frame False {
              }
              frame True {
                n3020 = property on="square matrix" class="Bool (strict)"("Value"=TRUE ("square matrix")) -> ()  [unwired: 2 in, 2 out]
                n3021 = property on="Square pixels" class="Bool (strict)"("Value"=FALSE ("square matrix")) -> ()  [unwired: 2 in, 2 out]
              }
            }
          }
          event "up", "downright", "down", "downleft", "right", "left", "upright", "upleft": Value Change {
            n3022 = event-data() -> ()  [unwired: 1 in, 6 out]
            n3023 = local read "downright"() -> (w6244:bool)
            n3024 = local read "downleft"() -> (w6246:bool)
            n3025 = local read "upright"() -> (w6242:bool)
            n3026 = local read "upleft"() -> (w6240:bool)
            n3027 = local read "down"() -> (w6245:bool)
            n3028 = local read "right"() -> (w6243:bool)
            n3029 = local read "left"() -> (w6247:bool)
            n3030 = local read "up"() -> (w6241:bool)
            n3031 = Compound Arithmetic op=OR(w6240, w6241, w6242, w6243, w6244, w6245, w6246, w6247) -> (w6239:bool)
            n3032 = case shown="True" w6239 {
              frame False {
              }
              frame True {
                n3033 = stacked-sequence {
                  frame #0 {
                    n3034 = local read "downright"() -> (w6249:bool)
                    n3035 = local read "downleft"() -> (w6251:bool)
                    n3036 = local read "BigSmall"() -> (w6248:bool)
                    n3037 = local read "upright"() -> (w6253:bool)
                    n3038 = local read "upleft"() -> (w6256:bool)
                    n3039 = local read "down"() -> (w6252:bool)
                    n3040 = local read "right"() -> (w6254:bool)
                    n3041 = local read "left"() -> (w6250:bool)
                    n3042 = local read "up"() -> (w6255:bool)
                    n3043 = call "movestageparams.vi"("command"="get") -> ("Params out"=w6259:T20)  [unwired: 1 in]
                    n3044 = Bundle By Name(cluster=w6259, "upleft"=w6256, "up"=w6255, "upright"=w6253, "right"=w6254, "downright"=w6249, "down"=w6252, "downleft"=w6251, "left"=w6250, "Bigsmall"=w6248) -> (w6260:T20)
                    n3045 = call "movestageparams.vi"("Params in"=w6260, "command"="set") -> ()  [unwired: 1 out]
                  }
                  frame #1 {
                    n3046 = disable-structure shown="Disabled" {
                      frame Disabled {
                        n3047 = call "configuration.vi"("command"="get") -> ("config out"=w6263:T11)  [unwired: 2 in, 1 out]
                        n3048 = in-place {
                          n3049 = in-place-cluster #45(w6263) -> ()  [unwired: 2 out]
                          n3050 = in-place-cluster #45("StageL"="StageL", "StageS"="StageS") -> (w6261:T11)
                        }
                        n3051 = call "configuration.vi"("config in"=w6261, "command"="set") -> ()  [unwired: 1 in, 2 out]
                      }
                      frame Enabled {
                      }
                    }
                  }
                  frame #2 {
                    n3052 = call "movestage.vi"() -> ()  [unwired: 12 in]
                  }
                  frame #3 {
                    w6267 = FALSE ("OK Button")
                    w6268 = FALSE ("OK Button")
                    n3053 = property on="down" class="Bool (strict)"("Value"=w6268) -> ()  [unwired: 2 in, 2 out]
                    n3054 = property on="up" class="Bool (strict)"("Value"=w6268) -> ()  [unwired: 2 in, 2 out]
                    n3055 = property on="right" class="Bool (strict)"("Value"=w6268) -> ()  [unwired: 2 in, 2 out]
                    n3056 = property on="left" class="Bool (strict)"("Value"=w6268) -> ()  [unwired: 2 in, 2 out]
                    n3057 = property on="upright" class="Bool (strict)"("Value"=w6267) -> ()  [unwired: 2 in, 2 out]
                    n3058 = property on="downleft" class="Bool (strict)"("Value"=w6267) -> ()  [unwired: 2 in, 2 out]
                    n3059 = property on="downright" class="Bool (strict)"("Value"=w6267) -> ()  [unwired: 2 in, 2 out]
                    n3060 = property on="upleft" class="Bool (strict)"("Value"=w6267) -> ()  [unwired: 2 in, 2 out]
                  }
                }
              }
            }
          }
          event "finite samples": Value Change {
            n3061 = event-data() -> ("NewVal"=w6269:bool)  [unwired: 1 in]
            n3062 = flat-sequence {
              tunnel: w6269 -> [w6270]
              frame #0 {
                n3063 = case shown="True" w6270 {
                  frame False {
                    w6271 = FALSE ("wavdet")
                    n3064 = property on="continuous" class="Bool (strict)"("Value"=TRUE ("continuous for display")) -> ()  [unwired: 2 in, 2 out]
                    n3065 = property on="wavdet" class="Bool (strict)"("Value"=w6271) -> ()  [unwired: 2 in, 2 out]
                    n3066 = property on="save\ndata" class="Bool (strict)"("Value"=w6271) -> ()  [unwired: 2 in, 2 out]
                    n3067 = property on="# of frames" class="DigNum (strict)"("DisabledEnum"=T7."Disabled and Grayed Out" ("Disabled")) -> ()  [unwired: 2 in, 2 out]
                    n3068 = property on="save\ndata" class="Bool (strict)"("DisabledEnum"=T7."Disabled and Grayed Out" ("Disabled")) -> ()  [unwired: 2 in, 2 out]
                    "Save tab" <- enum32{"withsave", "withoutsave"}."withsave" ("Save tab")
                  }
                  frame True {
                    w6278 = FALSE ("continuous for display")
                    n3069 = property on="continuous" class="Bool (strict)"("Value"=w6278) -> ()  [unwired: 2 in, 2 out]
                    n3070 = property on="wavdet" class="Bool (strict)"("Value"=w6278) -> ()  [unwired: 2 in, 2 out]
                    n3071 = local write "Save tab"(enum32{"withsave", "withoutsave"}."withsave" ("Save tab")) -> ()
                    n3072 = property on="save\ndata" class="Bool (strict)"("DisabledEnum"=T7."Enabled" ("Disabled")) -> ()  [unwired: 2 in, 2 out]
                    n3073 = property on="save\ndata" class="Bool (strict)"("Value"=TRUE ("save\ndata")) -> ()  [unwired: 2 in, 2 out]
                    n3074 = property on="# of frames" class="DigNum (strict)"("DisabledEnum"=T7."Enabled" ("Disabled")) -> ()  [unwired: 2 in, 2 out]
                  }
                }
              }
              frame #1 {
                n3075 = local read "finite samples"() -> (w6287:bool)
                n3076 = local read "continuous"() -> (w6286:bool)
                n3077 = local read "wavdet"() -> (w6285:bool)
                n3078 = call "2pparameters.vi"("command"="get") -> ("params out"=w6281:T10)  [unwired: 1 in]
                n3079 = Bundle By Name(cluster=w6281, "finite"=w6287, "cont"=w6286, "wavdet"=w6285) -> (w6284:T10)
                n3080 = call "2pparameters.vi"("Params in"=w6284, "command"="set") -> ()  [unwired: 1 out]
              }
            }
          }
          event "continuous": Value Change {
            n3081 = event-data() -> ("NewVal"=w6288:bool)  [unwired: 1 in]
            n3082 = flat-sequence {
              tunnel: w6288 -> [w6289]
              frame #0 {
                n3083 = case shown="True" w6289 {
                  frame False {
                    n3084 = property on="finite samples" class="Bool (strict)"("Value"=TRUE ("finite samples for recording")) -> ()  [unwired: 2 in, 2 out]
                    n3085 = property on="save\ndata" class="Bool (strict)"("Value"=TRUE ("save\ndata")) -> ()  [unwired: 2 in, 2 out]
